vi "monitor wavelength change.vi"(6 "Ls1 wav cancel":refnum<vi>, 7 "Actions":T1(ring), 8 "error in (no error)":errorcluster, 9 "new val":dbl, 10 "Old val":dbl, 11 "CtlRef":refnum<vi>) -> (0 "error out":errorcluster, 2 "time stamp":timestamp, 3 "Boolean":bool)   [LabVIEW 2017]
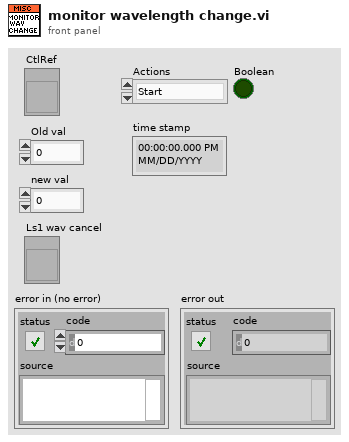
[diagram p1: front panel]
types:
  T1 = enum16{"Start", "Display status", "Monitor", "Cancel", "Stop"}
  T2 = enum8{"Enabled", "Disabled", "Disabled and Grayed Out"}
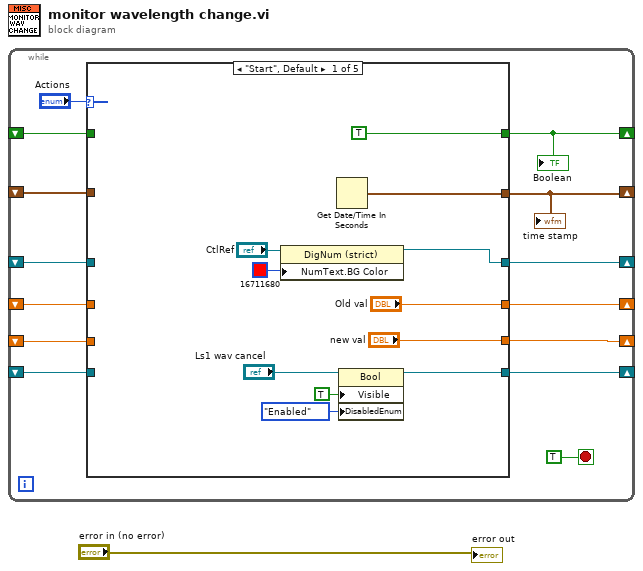
[diagram p0: block diagram]
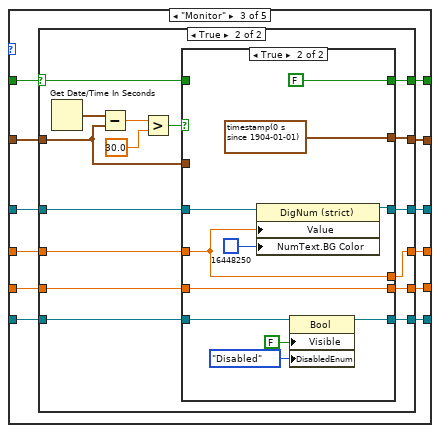
[diagram p3: hidden frame]
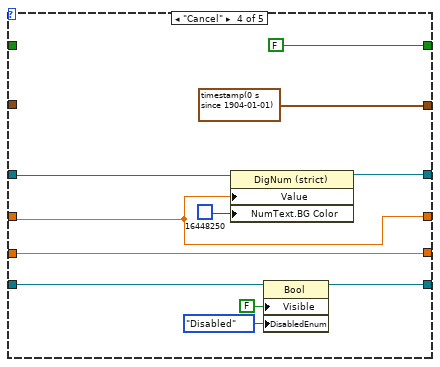
[diagram p6: hidden frame]
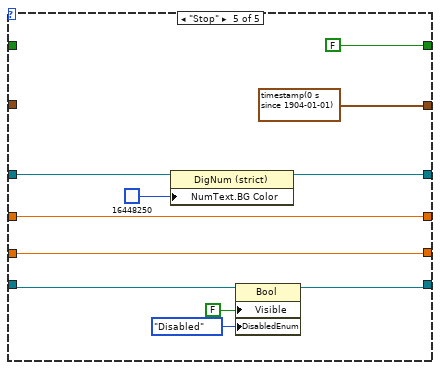
[diagram p7: hidden frame]
diagram:
  n1 = while {
    shift-right: [w14] -> _
    shift-left: _ -> [w13]
    shift-right: [w12] -> _
    shift-left: _ -> [w11]
    shift-right: [w9] -> _
    shift-left: _ -> [w8]
    shift-right: [w7] -> _
    shift-left: _ -> [w5]
    shift-right: [w6] -> _
    shift-left: _ -> [w4]
    shift-right: [w3] -> _
    shift-left: _ -> [w2]
    stop <- TRUE stop-if-true
    n2 = case shown="\"Start\", Default" "Actions" {
      tunnel: [w25 w31 w40 timestamp(0 s since 1904-01-01) ("time stamp") timestamp(0 s since 1904-01-01) ("time stamp")] -> w14
      tunnel: w13 -> [_ w31 w43 _ _]
      tunnel: [TRUE w32 w41 FALSE FALSE] -> w12
      tunnel: w11 -> [_ w32 w44 _ _]
      tunnel: [w20 w30 w39 w88 w100] -> w9
      tunnel: w8 -> [_ w30 w42 w89 w101]
      tunnel: ["Old val" w29 w37 w87 w103] -> w7
      tunnel: ["new val" w28 w35 w86 w102] -> w6
      tunnel: w5 -> [_ w29 w38 w87 w103]
      tunnel: w4 -> [_ w28 w36 w86 w102]
      tunnel: [w17 w27 w33 w84 w96] -> w3
      tunnel: w2 -> [_ w27 w34 w85 w97]
      frame "Start", Default {
        n3 = property class="DigNum (strict)"(reference="CtlRef", "NumText.BG Color"=u32 16711680) -> (reference out=w20:refnum<vi>)  [unwired: 1 in, 1 out]
        n4 = Get Date/Time In Seconds() -> (seconds since 1Jan1904=w25:timestamp)
        n5 = property class="Bool"(reference="Ls1 wav cancel", "Visible"=TRUE, "DisabledEnum"=T2."Enabled" ("Disabled")) -> (reference out=w17:refnum<vi>)  [unwired: 1 in, 1 out]
      }
      frame "Display status" {
      }
      frame "Monitor" {
        n6 = case shown="True" w44 {
          selector: w44 -> [w50 w61]
          tunnel: w43 -> [w49 w58]
          tunnel: w42 -> [w48 w62]
          tunnel: [w50 w60] -> w41
          tunnel: [w49 w59] -> w40
          tunnel: [w48 w57] -> w39
          tunnel: w38 -> [w47 w56]
          tunnel: [w47 w55] -> w37
          tunnel: w36 -> [w46 w54]
          tunnel: [w46 w53] -> w35
          tunnel: w34 -> [w45 w52]
          tunnel: [w45 w51] -> w33
          frame False {
          }
          frame True {
            n7 = Get Date/Time In Seconds() -> (seconds since 1Jan1904=w66:timestamp)
            n8 = Subtract(x=w66, y=w58) -> (x-y=w65:dbl)
            n9 = Greater?(x=w65, y=30.0) -> (0:w63:bool)
            n10 = case shown="True" w63 {
              tunnel: w62 -> [w70 w81]
              tunnel: w61 -> [w72 _]
              tunnel: [w72 FALSE] -> w60
              tunnel: [w71 timestamp(0 s since 1904-01-01) ("time stamp")] -> w59
              tunnel: w58 -> [w71 _]
              tunnel: [w70 w80] -> w57
              tunnel: w56 -> [w69 w78]
              tunnel: [w69 w78] -> w55
              tunnel: w54 -> [w68 w79]
              tunnel: [w68 w79] -> w53
              tunnel: w52 -> [w67 w75]
              tunnel: [w67 w76] -> w51
              frame False {
              }
              frame True {
                n11 = property class="DigNum (strict)"(reference=w81, "Value"=w78, "NumText.BG Color"=u32 16448250) -> (reference out=w80:refnum<vi>)  [unwired: 1 in, 1 out]
                n12 = property class="Bool"(reference=w75, "Visible"=FALSE, "DisabledEnum"=T2."Disabled" ("Disabled")) -> (reference out=w76:refnum<vi>)  [unwired: 1 in, 1 out]
              }
            }
          }
        }
      }
      frame "Cancel" {
        n13 = property class="DigNum (strict)"(reference=w89, "Value"=w87, "NumText.BG Color"=u32 16448250) -> (reference out=w88:refnum<vi>)  [unwired: 1 in, 1 out]
        n14 = property class="Bool"(reference=w85, "Visible"=FALSE, "DisabledEnum"=T2."Disabled" ("Disabled")) -> (reference out=w84:refnum<vi>)  [unwired: 1 in, 1 out]
      }
      frame "Stop" {
        n15 = property class="DigNum (strict)"(reference=w101, "NumText.BG Color"=u32 16448250) -> (reference out=w100:refnum<vi>)  [unwired: 1 in, 1 out]
        n16 = property class="Bool"(reference=w97, "Visible"=FALSE, "DisabledEnum"=T2."Disabled" ("Disabled")) -> (reference out=w96:refnum<vi>)  [unwired: 1 in, 1 out]
      }
    }
    "Boolean" <- w12
    "time stamp" <- w14
  }
  "error out" <- "error in (no error)"
